vi "Get Firings.vi"(11 "Cerebellum in":refnum<class "Cerebellum.lvclass">) -> (0 "No N":i32[](array[numeric]), 1 "Currents Left":dbl[](array[numeric]), 2 "Currents Right":dbl[](array[numeric]), 3 "Cerebellum out":refnum<class "Cerebellum.lvclass">)   [LabVIEW 2016, in "Cerebellum.lvclass"]
uses:
  Cerebellum.lvclass
  Cerebellum.lvclass/Cerebellum.ctl
  AER/AER.lvclass/AER.ctl
  AER/AER.lvclass
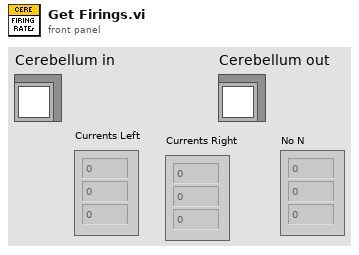
[diagram p1: front panel]
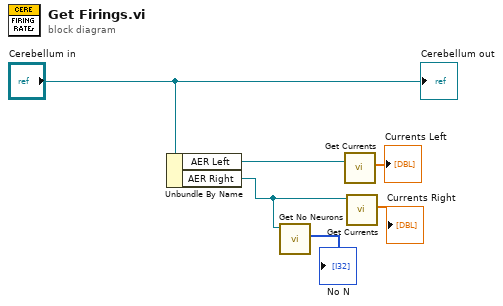
[diagram p0: block diagram]
diagram:
  n1 = Unbundle By Name("Cerebellum in") -> ("AER Left"=w5:refnum<class "AER.lvclass">, "AER Right"=w2:refnum<class "AER.lvclass">)
  n2 = call "Get No Neurons.vi"("AER in"=w2) -> ("No N"=→"No N":i32[])  [unwired: 9 in, 1 out]
  n3 = call "Get Currents.vi"("AER in"=w5) -> ("Currents"=→"Currents Left":dbl[])  [unwired: 8 in, 2 out]
  n4 = call "Get Currents.vi"("AER in"=w2) -> ("Currents"=→"Currents Right":dbl[])  [unwired: 8 in, 2 out]
  "Cerebellum out" <- "Cerebellum in"
